vi "Close.vi"(7 "Version":i32, 8 "error in (no error)":errorcluster caption="entrée d'erreur (pas d'erreur)") -> (0 "error out":errorcluster, 3 "Open Out":string)   [LabVIEW 2012, in "TiffLib.lvlib"]
uses:
  TiffLib.lvlib
  Librairies/TiffLib_v1/TiffLib_v1.lvlib
  Librairies/TiffLib_v2/TiffLib_v2.lvlib
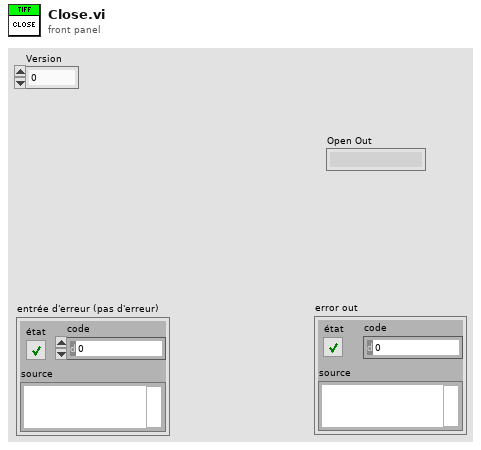
[diagram p1: front panel]
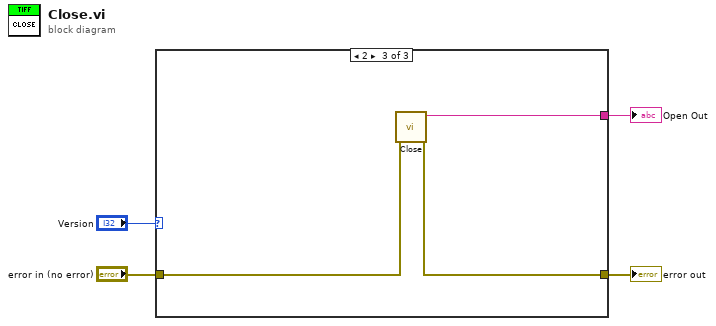
[diagram p0: block diagram]
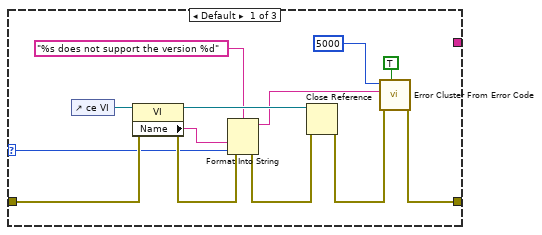
[diagram p2: hidden frame]
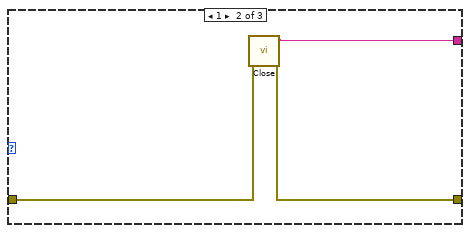
[diagram p3: hidden frame]
diagram:
  n1 = case shown="2" "Version" {
    selector: "Version" -> [w10 _ _]
    tunnel: [_ w18 w23] -> w3
    tunnel: "error in (no error)" -> [w13 w20 w21]
    tunnel: [w17 w19 w22] -> w1
    frame Default {
      n2 = control-ref of="ce VI"() -> (w14:refnum<vi>)
      n3 = property class="VI"(reference=w14, error in=w13) -> (reference out=w9:refnum<vi>, error out=w12:errorcluster, "Name"=w11:string)
      n4 = Format Into String(format string="%s does not support the version %d" ("chaîne de format"), error in=w12, w11, w10) -> (resulting string=w6:string, error out=w8:errorcluster)  [unwired: 1 in]
      n5 = Close Reference(reference=w9, error in (no error)=w8) -> (error out=w7:errorcluster)
      n6 = call <vilib>:"Error Cluster From Error Code.vi"("show call chain? (False)"=TRUE, "error in (no error)"=w7, "error message (\"\")"=w6, "error code (0)"=5000) -> ("error out"=w17:errorcluster)  [unwired: 5 in]
    }
    frame 1 {
      n7 = call "Close.vi"("error in (no error)"=w20) -> ("error out"=w19:errorcluster, "Close Out"=w18:string)  [unwired: 9 in]
    }
    frame 2 {
      n8 = call "Close.vi"("error in (no error)"=w21) -> ("error out"=w22:errorcluster, "Close Out"=w23:string)  [unwired: 9 in]
    }
  }
  "Open Out" <- w3
  "error out" <- w1
